vi "AlliGator 1-Exp + IRF Fit v2.vi"(0 "Decay":cluster{"t Array":dbl[], "Data Array":dbl[]}, 1 "Optimal Offset Selection Criterion":T2, 5 "IRF":cluster{"t Array":dbl[], "IRF Array":dbl[]}, 7 "Fit Options":T12={"Show Fit Residuals"=TRUE, "Fit Model"=enum."1-Exponential", "Residual Type"=enum."Standard", "Max Decay Percentile"=0.0, "Min Decay Percentile"=0.0, "Show Full Decay"=TRUE, "Weights"=enum."Unweighted", "Fitting Method"=enum."Least Square", "Compute Parameter Uncertainties"=TRUE, "Periodic Boundaries"=TRUE, "Model Calculation"=enum."Simulation", "Period"=1.2500000000000001e-08, "Termination Criteria"={"Max Iterations"=1000, "Max Function Calls"=0, "Max Time"=1000.0, "Function Tolerance"=1e-06, "Parameter Tolerance"=1e-06, "Gradient Tolerance"=0.0, "Min Lambda"=1e-06, "Max Lambda"=1e-06, "Initial Tick Count"=0}, "Offset Resolution"=1.2500000000000001e-08, "Use Local IRF"=TRUE, "Fitting Algorithm"=enum."Levenberg-Marquardt", "Show Confidence Interval "=TRUE, "Confidence Level"=95.0} {"Confidence Level" min=0.0 max=100.0; "Offset Resolution" min=0.0; "Period" min=0.0; "Min Decay Percentile" min=0.0 max=1.0; "Max Decay Percentile" min=0.0 max=100.0}, 11 "error in (no error)":errorcluster, 12 "parameter bounds":T11) -> (4 "Fit Plots":T1, 8 "Fit Output":T4={"best nonlinear fit"=[], "best fit parameters"=[], "R^2"=0.0, "RMSE"=0.0, "error out"={"status"=FALSE, "code"=0, "source"=""}, "Fitting Method"=enum."Least Square", "number of function calls"=0, "number of iterations"=0, "covariance"=[], "Chi 2"=0.0, "DOF"=0, "Fit Convergence Criterion"=enum."Continue", "Fitting Algorithm"=enum."Levenberg-Marquardt", "Weighted Fit"=enum."Unweighted", "Gradient"=0.0, "|Delta Chi 2|"=0.0, "|Delta Chi 2|/Chi 2"=0.0, "Max |Delta a| /|a|"=0.0, "Lambda"=-1.0, "RSS"=0.0, "AIC"=0.0, "BIC"=0.0, "Max number of function calls"=0, "Max number of iterations"=0, "IRF"={"X Array"=[], "Y Array"=[]}, "IRF Normalization Factor"=0.0, "Decay Normalization Factor"=0.0, "Number of offset fits"=0, "Weighted Chi2"=-1.0, "Unweighted Chi2"=-1.0}, 10 "Delta Best Fit Parameters":dbl[](array[numeric]), 13 "Guess Parameters Options":T3=enum."User-provided (normalized)", 14 "Guess Parameters":dbl[](array[numeric]), 15 "error out":errorcluster)   [LabVIEW 2021, in "AlliGator Decay Fit.lvlib"]
doc: "Legacy code for 1-Exp decay fit."
uses:
  AlliGator Decay Fit.lvlib
  Fits/IRF(X)PSED/Decay Fit Options v4.ctl
  Fits/Decay Convolution/Decay Model.ctl
  Fits/Residual Type.ctl
  Fits/IRF(X)PSED/Fit Weights Type v2.ctl
  Fits/Non-linear Fitting Method v2.ctl
  Fits/Fit Calculation Method.ctl
  Fits/Non-linear Fitting Algorithm.ctl
  Fits/Non-linear Fit Output v4.ctl
  Fits/Nonlinear Fit Method.ctl
  <vilib>/Analysis/Matrix/Datatypes/RealMatrix.ctl
  Fits/Convergence Criteria.ctl
  Graphs/XY Graph/XY Graph Plot Data.ctl
  AlliGator Guess Parameters Options.ctl
  Fits/Optimal Offset Selection Criterion.ctl
  Fits/Fit Plots.ctl
  Settings/AlliGator Settings List.ctl
  Fits/Decay Convolution/Fit Control Data.ctl
  Globals, Variables, Constants/AlliGator Variables List.ctl
  Fits/Decay Convolution/LM model function and gradient (1-Exp, Convolved) v2.vi
  Phasor/Phasor Abort Parallel Computation.vi
  Fits/Decay Convolution/LM model function and gradient (1-Exp, Convolved, Periodic) v3.vi
  Fits/Decay Convolution/LM model function and gradient (1-Exp, Gated, Periodic).vi
  <vilib>/Utility/error.llb/Error Cluster From Error Code.vi
  Fits/Abort Fit Global.vi
  <vilib>/ErrorRing/Error Ring.xnode
  Time/Time.lvlib
  Fits/Fits.lvlib
  Settings/AlliGator Settings.lvlib
  Phasor/Phasor.lvlib
  Globals, Variables, Constants/AlliGator Globals, Variables & Constants.lvlib
  Error/Error.lvlib
  Graphs/XY Graph/XY Graph Add-Ons.lvlib
  <vilib>/Analysis/Matrix/NI_Matrix.lvlib
panel:
  out "CPU (s)":dbl
  out "XY Graph":T17(graph)
  # "Offset\nBaseline\nAmplitude\nLifetime"
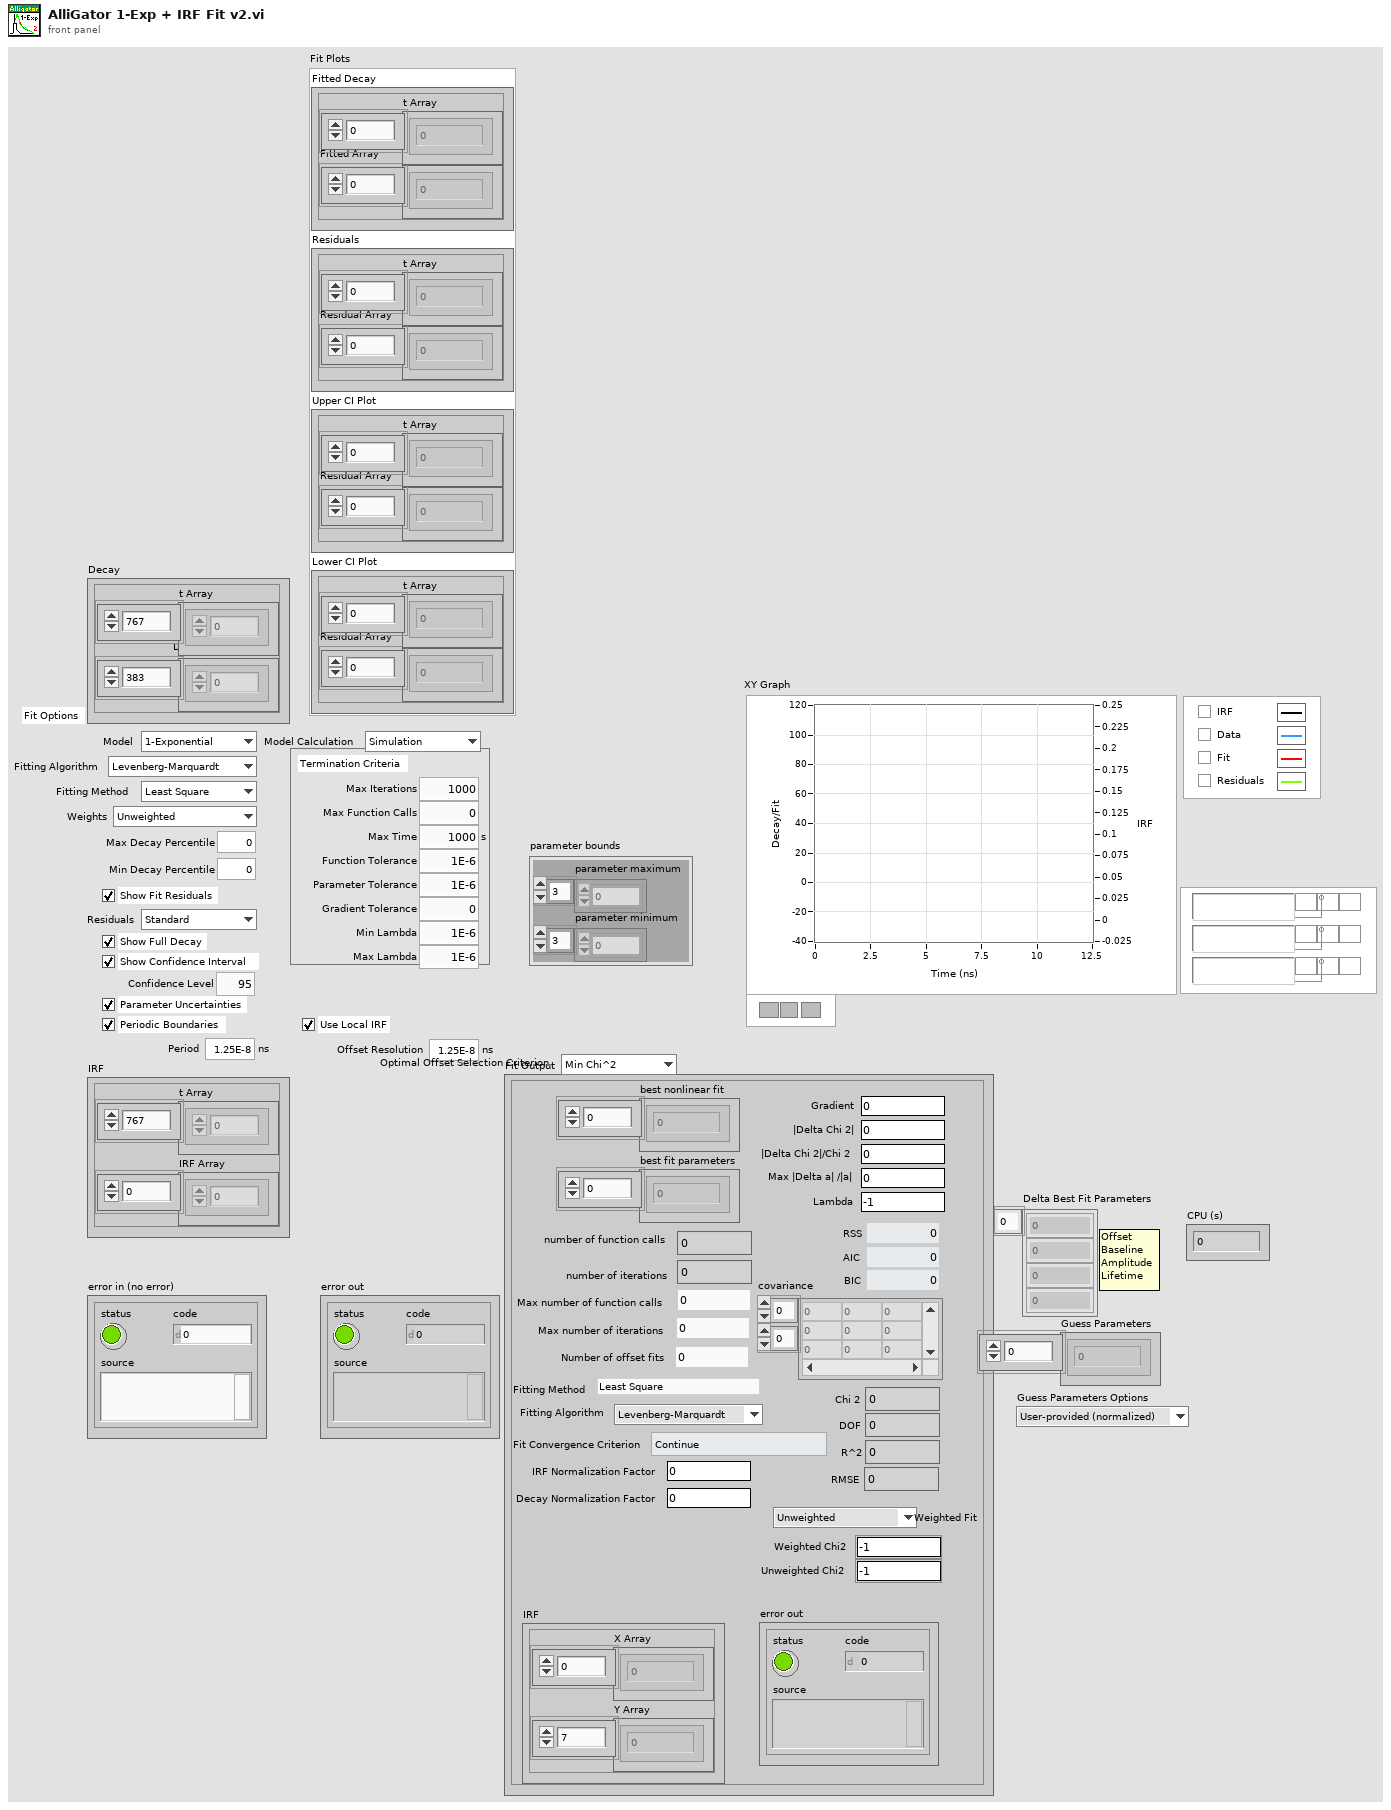
[diagram p1: front panel]
types:
  T1 = typedef "Fits.lvlib/Fit Plots.ctl" = cluster{"Fitted Decay":cluster{"t Array":dbl[], "Fitted Array":dbl[]}, "Residuals":cluster{"t Array":dbl[], "Residual Array":dbl[]}, "Upper CI Plot":cluster{"t Array":dbl[], "Residual Array":dbl[]}, "Lower CI Plot":cluster{"t Array":dbl[], "Residual Array":dbl[]}}
  T2 = typedef "Fits.lvlib/Optimal Offset Selection Criterion.ctl" = enum16{"Min Chi^2", "Max R^2"}
  T3 = typedef "AlliGator Decay Fit.lvlib/AlliGator Guess Parameters Options.ctl" = enum16{"Numerically estimated", "User-provided", "User-provided (normalized)", "Last valid fitted parameters"}
  T4 = typedef "Fits.lvlib/Non-linear Fit Output v4.ctl" = cluster{"best nonlinear fit":dbl[], "best fit parameters":dbl[], "R^2":dbl, "RMSE":dbl, "error out":errorcluster, "Fitting Method":T5, "number of function calls":i32, "number of iterations":i32, "covariance":T6, "Chi 2":dbl, "DOF":i32, "Fit Convergence Criterion":T7, "Fitting Algorithm":T8, "Weighted Fit":T9, "Gradient":dbl, "|Delta Chi 2|":dbl, "|Delta Chi 2|/Chi 2":dbl, "Max |Delta a| /|a|":dbl, "Lambda":dbl, "RSS":dbl, "AIC":dbl, "BIC":dbl, "Max number of function calls":i32, "Max number of iterations":i32, "IRF":T10, "IRF Normalization Factor":dbl, "Decay Normalization Factor":dbl, "Number of offset fits":i32, "Weighted Chi2":dbl, "Unweighted Chi2":dbl}
  T5 = typedef "Fits.lvlib/Nonlinear Fit Method.ctl" = enum16{"Least Square", "Least Absolute Residual", "Bisquare", "MLE"}
  T6 = typedef "NI_Matrix.lvlib/RealMatrix.ctl" = dbl[][]
  T7 = typedef "Fits.lvlib/Convergence Criteria.ctl" = enum16{"Continue", "Tolerances Exceeded", "Max Time Exceeded", "Max Iterations Exceeded", "Max Function Evaluations Exceeded", "Scale Range Exceeded"}
  T8 = typedef "Fits.lvlib/Non-linear Fitting Algorithm.ctl" = enum16{"Levenberg-Marquardt", "Trust-Region Dogleg"}
  T9 = typedef "Fits.lvlib/Fit Weights Type v2.ctl" = enum16{"Unweighted", "1/Variance (Neyman)", "1/Variance (Pearson)", "Best of All"}
  T10 = typedef "XY Graph Add-Ons.lvlib/XY Graph Plot Data.ctl" = cluster{"X Array":dbl[], "Y Array":dbl[]}
  T11 = cluster{"parameter minimum":dbl[], "parameter maximum":dbl[]}
  T12 = typedef "Fits.lvlib/Decay Fit Options v4.ctl" = cluster{"Show Fit Residuals":bool, "Fit Model":T13, "Residual Type":T14, "Max Decay Percentile":dbl, "Min Decay Percentile":dbl, "Show Full Decay":bool, "Weights":T9, "Fitting Method":T15, "Compute Parameter Uncertainties":bool, "Periodic Boundaries":bool, "Model Calculation":T16, "Period":dbl[unit], "Termination Criteria":cluster{"Max Iterations":i32, "Max Function Calls":i32, "Max Time":dbl[unit], "Function Tolerance":dbl, "Parameter Tolerance":dbl, "Gradient Tolerance":dbl, "Min Lambda":dbl, "Max Lambda":dbl, "Initial Tick Count":u32}, "Offset Resolution":dbl[unit], "Use Local IRF":bool, "Fitting Algorithm":T8, "Show Confidence Interval ":bool, "Confidence Level":dbl}
  T13 = typedef "Fits.lvlib/Decay Model.ctl" = enum16{"1-Exponential", "2-Exponentials"}
  T14 = typedef "Fits.lvlib/Residual Type.ctl" = enum16{"Standard", "Normalized", "Reduced"}
  T15 = typedef "Fits.lvlib/Non-linear Fitting Method v2.ctl" = enum16{"Least Square", "Least Absolute Residual", "Bisquare", "MLE", "-", "Best of All"}
  T16 = typedef "Fits.lvlib/Fit Calculation Method.ctl" = enum16{"Simulation", "Convolution", "Integration"}
  T17 = cluster{"t Array":dbl[], "best nonlinear fit":dbl[]}[]
  T18 = typedef "AlliGator Settings.lvlib/AlliGator Settings List.ctl" = enum16{"GUI:Visible Settings Tab", "GUI:Last Run Version", "Source Image:Use Image Histogram for Contrast", "Source Image:Low Count Pixels Rejection Options", "Source Image:High Count Pixels Rejection Options", "Source Image:Use Image Brightness", "Source Image:Blend Overlay with Image Background", "Source Image:Use Fixed ROI Diameter", "Source Image:ROI Diameter", "Source Image:ROI Center Color", "Source Image:Peak Threshold", "Source Image:Intensity Threshold", "Source Image:Image Binning Options", "Source Image:Image Smoothing Options", "Source Image:Image Histogram Active", "Source Image:Invert Binary Mask", "Source Image:Hot Pixel Removal", "Source Image:Overlay Analyzed ROI Center", "Source Image:Auto-Adjust Contrast", "Source Image:Histogram Lower Percentile", "Source Image:Histogram Upper Percentile", "Source Image:Save Source Image", "Source Image:Scale Bar Options", "Source Image:Image Resolution (Pixel Size)", "Source Image:Flatfield Correction", "Source Image:Show Dead Left Columns Correction", "Source Image:Dead Left Columns Correction", "Source Image:Image Pre-Processing Operations Order", "Source Image:Overlay ROI Median", "Source Image:Median Overlay Color", "Data Information:Gate Width", "Data Information:Nanotime Gate Separation", "Data Information:Macrotime Gate Separation", "Data Information:Gate Step", "Data Information:# Gates", "Data Information:Gate Image Exposure", "Data Information:Gate Image Integration", "Data Information:Gates to Skip", "Data Information:Gates to Keep", "Data Information:Define Gates to", "Data Information:Channel Name", "Data Information:Available Channel Names", "Data Information:Channel Arithmetic", "Data Information:Background File Subtraction", "Data Information:Background File", "Data Information:Background Scaling Factor", "Data Information:Background Pile-up Correction", "Data Information:Background Pixel Well Capacity", "Data Information:Laser Period", "Data Information:SYNC Period", "Data Information:Pile-up Correction", "Data Information:Pixel Well Capacity", "Data Information:Dataset Scaling Factor", "Fluorescence Decay_Decay Pre-Processing:Reverse Gates", "Fluorescence Decay_Decay Pre-Processing:Verbose Decay Pre-Processing", "Fluorescence Decay_Decay Pre-Processing:Use Decay Pre-Processing", "Fluorescence Decay_Decay Pre-Processing:Background Subtraction", "Fluorescence Decay_Decay Pre-Processing:Background Definition Range", "Fluorescence Decay_Decay Pre-Processing:Baseline Subtraction Method", "Fluorescence Decay_Decay Pre-Processing:Decay Pre-Processing Operations Order", "Fluorescence Decay_Decay Pre-Processing:Smoothing Parameter", "Fluorescence Decay_Decay Pre-Processing:Shift Decay", "Fluorescence Decay_Decay Pre-Processing:Decay Shift Parameters", "Fluorescence Decay_Decay Pre-Processing:Fold Decay", "Fluorescence Decay_Decay Pre-Processing:# Folds", "Fluorescence Decay_Decay Pre-Processing:1-Normalize Decay", "Fluorescence Decay_Decay Pre-Processing:[0-1]-Normalize Decay", "Fluorescence Decay_Decay Pre-Processing:Smoothen Decay", "Fluorescence Decay_Decay Pre-Processing:Extrapolate Decay", "Fluorescence Decay_Decay Pre-Processing:Use Periodicity", "Fluorescence Decay_Decay Pre-Processing:Use Cursors", "Fluorescence Decay_Decay Pre-Processing:Tail Fraction", "Fluorescence Decay_Decay Pre-Processing:Head Fraction", "Fluorescence Decay_Decay Pre-Processing:Additional Points", "Fluorescence Decay_Decay Pre-Processing:Straighten Decay", "Fluorescence Decay_Decay Pre-Processing:Constant Background", "Fluorescence Decay_Decay Pre-Processing:Pixel-Normalize Decay", "Fluorescence Decay_Advanced Analysis:Extract IRF instead of Decay", "Fluorescence Decay_Advanced Analysis:IRF Extraction Options", "Fluorescence Decay_Advanced Analysis:IRF Optimization Options", "Fluorescence Decay_Advanced Analysis:Square Pulse Options", "Fluorescence Decay_Advanced Analysis:IRF Order", "Fluorescence Decay_Advanced Analysis:IRF Time Constants", "Fluorescence Decay_Advanced Analysis:Wavelet Analysis Options", "Fluorescence Decay_Advanced Analysis:Average Lifetime Options", "Fluorescence Decay_Fit Options:Fit Options", "Fluorescence Decay_Fit Options:Use Legacy Fitting Approach", "Fluorescence Decay_Fit Options:Use Data Information Laser Period", "Fluorescence Decay_Fit Parameters:Displayed Fit Parameters", "Fluorescence Decay_Fit Parameters:Fit Parameter Constraints", "Fluorescence Decay_Fit Parameters:Export Tabulated Results", "Fluorescence Decay_Fit Parameters:MLE Baseline Offset Type", "Fluorescence Decay_Fit Parameters:MLE Baseline Offset", "Fluorescence Decay_Fit Parameters:Guess Parameter Names", "Fluorescence Decay_Fit Parameters:Guess Parameter Values", "Fluorescence Decay_Fit Parameters:Guess Parameters Options", "Fluorescence Decay_Fit Parameters:Optimal Offset Selection Criterion", "Fluorescence Decay_Styles:Show Last Decay Only", "Fluorescence Decay_Styles:Decay Graph Color Array", "Fluorescence Decay:Decay Graph Active", "Fluorescence Decay Statistics:Min Peak Value", "Fluorescence Decay Statistics:Reject Low Decay Peak Pixels", "Fluorescence Decay Statistics:Reject High Decay Peak Pixels", "Fluorescence Decay Statistics:Max Peak Value", "Time Traces:Use File Timestamp", "Time Traces:Time Step", "Time Traces:Use Intensity Correction File", "Time Traces:Intensity Correction File", "Phasor Plot:Phasor Plot Smoothing Options", "Phasor Plot:Phasor Plot Size", "Phasor Plot:Phasor Plot Graphics Options", "Phasor Plot:Cumulative Phasor Plot", "Phasor Plot:Use Phasor Brightness", "Phasor Plot:Blend Overlay with Phasor Background", "Phasor Plot:Save Phasor Plot", "Phasor Plot:Show References", "Phasor Plot:Phasor Ratio Decay Range", "Phasor Plot:Exponential Fading", "Phasor Plot:Phasor Ratio Reference Colors", "Phasor Plot:Reference Radius", "Phasor Plot:Show Color Map Vertices", "Phasor Plot:Phasor Plot Active", "Phasor Plot:Phasor Ratio Color Map Type", "Phasor Plot:Phasor Ratio Color Map", "Phasor Plot:Phasor Ratio Display Range", "Phasor Plot:Selected Image ROI(s)", "Phasor Plot:All Image ROIs", "Phasor Plot:Selected Phasor Plot ROI(s)", "Phasor Plot:All Phasor Plot ROIs", "Phasor Plot:Phasor Ratio Color-Coded Quantity", "Phasor Plot:Store Phasor Harmonics", "Phasor Plot:Draw Reference Segment", "Phasor Plot:User-Defined Quantity", "Phasor Plot:Color Scale High Color", "Phasor Plot:Color Scale Low Color", "Phasor Plot:Intensity-weighted Phasor Plot", "Phasor Graph:Phasor Frequency", "Phasor Graph:Phasor Ratio Type", "Phasor Graph:Pixel-level Phasor Computation", "Phasor Graph:Save Phasor Graph", "Phasor Graph:Phasor Graph Active", "Phasor Graph:Phasor SDV Options", "Phasor Graph:Intensity-weighted Phasor Graph", "Phasor Graph:Define Shortest Lifetime as", "Phasor Calibration:Use Backup Calibration if needed", "Phasor Calibration:Backup Calibration Type", "Phasor Calibration:Calibration Type", "Phasor Calibration:Calibration Lifetime", "Phasor Calibration:Calibration Map Algorithm", "Single-Exponential Phasor Locus (SEPL):Gate Parameters", "Single-Exponential Phasor Locus (SEPL):User-defined Gate", "Single-Exponential Phasor Locus (SEPL):User-defined IRF", "Single-Exponential Phasor Locus (SEPL):Phasor Parameters", "Single-Exponential Phasor Locus (SEPL):Decay & IRF Parameters", "Single-Exponential Phasor Locus (SEPL):Display Parameters", "Lifetime Analysis:Decay Analysis Parameters", "Lifetime Analysis:Lifetime Map Active", "Plugins:Python Settings", "Miscellaneous:Verbose Mode", "Miscellaneous:Beep after Script", "Miscellaneous:Saved Image File Format", "Miscellaneous:Exported Gate Image Settings", "Miscellaneous:Include Loading in Timing", "Miscellaneous:Verbose Settings Mode", "Miscellaneous:Histogram Options", "Miscellaneous:Beep on Error", "Miscellaneous:# Logical Processors Used", "Miscellaneous:ROI Description Max Characters", "Miscellaneous:Verbose Error Mode", "Miscellaneous:Transparent Mask Color"}
  T19 = typedef "Fits.lvlib/Fit Control Data.ctl" = cluster{"IRF":T10, "Laser Period":dbl, "SYNC Period":dbl}
  T20 = typedef "Fits.lvlib/Decay Fit Parameters In List.ctl" = enum16{"Offset", "Baseline", "A_1", "tau_1", "A_2", "tau_2"}
  T21 = typedef "Fits.lvlib/Fit Results (statistics).ctl" = cluster{"Chi2/DOF":dbl, "R2":dbl, "RMSE":dbl, "Fitting Method":T15, "Fitting Algorithm":T8}
  T22 = typedef "AlliGator Globals, Variables & Constants.lvlib/AlliGator Variables List.ctl" = enum16{"---- GUI ----", "GUI:Initialization Status", "GUI:State Indicators Refnum", "GUI:Original AlliGator Menu Items", "GUI:Current Action Loop State", "GUI:Script in progress", "GUI:Playback", "GUI:Loop Playback", "GUI:Search ROI Used", "GUI:Search ROI", "Decay Graph Max Legend Size", "Intensity Graph Max Legend Size", "Decay Statistics Graph Max Legend Size", "Phasor Graph Max Legend Size", "Phasor Ratio Graph Max Legend Size", "Lifetime Graph Max Legend Size", "---- Files ----", "Files:Export Dataset Frames as Individual Files", "Files:Show Batch Export Help Balloons", "Files:Frames in Dataset", "Files:ptu File Frame Start Indices", "Files:Current Frame in Dataset", "Files:Current Frame Timestamp", "Files:Dataset Loaded", "Files:Dataset Metadata", "Files:Dataset Channel", "Files:Dataset Data Description", "Files:Background Dataset Metadata", "Files:Background Dataset Channel", "Files:Background Dataset Data Description", "Files:Background File Subtraction", "Files:Background File Path", "Files:Background File Pile-up Correction", "Files:Background File Pixel Well Capacity", "Files:Background File Scaling Factor", "Files:Current Dataset Load Settings", "Files:Dataset Path", "Files:ICCD-specific Information", "Files:Macrotime Gate Separation", "------ Python Plugins ------", "Python Plugins:Information", "Python Plugins:Python Session", "Python Plugins:Valid Python Session?", "---- Source Image ----", "Source Image:ROIs", "Source Image:Current ROI", "Source Image:ROI Event Refnum", "X_Source Image:Display Range", "X_Source Image:Palette Information", "X_Source Image:Type of Displayed Image", "X_Time Gate Slider", "Source Image:Palette List", "Source Image:Scale", "Source Image:ROI Overlay Color", "Source Image:Overlay to Erase", "Source Image:Is Displayed Image Accumulated", "Source Image:White Light Image Modified", "Source Image:Mask Image Modified", "---- Image Profile Window ----", "Image Profile:Window Event Refnum", "Image Profile:IntensityType", "Image Profile:Intensity Average Type", "Image Profile:Intensity-weighted SDV", "Image Profile:Box Profile Type", "Image Profile:Window Open", "Image Profile:Plotted Fit Parameter", "------ Phasor Graph -------", "Phasor Graph:Show Line", "---- Phasor Plot ---", "Phasor Plot:Parameters Changed", "Phasor Plot:FLI Dataset Modified since last Calculation", "Phasor Harmonics Data", "Selected Phasor Harmonics", "Phasor Harmonic Manager Event Refnum", "Phasor Plot:ROIs", "Phasor Plot:Current ROI", "Phasor Plot:ROI Event Refnum", "Phasor Plot:Image Reference Points", "Phasor Plot:Computed", "Phasor Plot:Palette Information", "Phasor Plot:Palette List", "Phasor Plot:Phasor Ratio Palette Information", "Phasor Plot:Phasor Ratio Palette List", "Phasor Plot:Image Scale", "Phasor Plot:Image Overlay to Erase", "Phasor Plot:Image Elements to Update", "Phasor Plot:Current Calculation Parameters", "Phasor Plot:Current Calibration Options", "Phasor Plot:Reset Cumulated Phasor Plot", "Phasor Plot:Reference 1", "Phasor Plot:Lifetime Reference 1", "Phasor Plot:Reference 1 Frequency", "Phasor Plot:Reference 2", "Phasor Plot:Lifetime Reference 2", "Phasor Plot:Reference 2 Frequency", "---- Decay Analysis ----", "Number of Selected Decays to Fit", "LS Fit Results", "LAR Fit Results", "BS Fit Results", "Last Decay Max - Min", "Best Fit Parameters", "Best Fit Parameter Names", "Actual Size X", "Actual Size Y", "Binning X", "Binning Y", "Actual # Gates", "Dataset Number", "Gates to...", "Gates Skipped", "Gates to keep", "Gate Step", "Gate Separation", "Reversed Gates", "Pile-up Correction", "Pixel Well Capacity", "Background Subtracted", "Background Subtraction Method", "Background Definition Range", "Background File (deprecated)", "Number of Dataset Accumulated", "Array of Accumulated Dataset Paths", "Do Averaged Datasets", "Destination File Path", "Process Plot Target", "Use 1/D as Phasor Frequency", "---- Decay Fit Parameter Map -----", "Decay Fit Parameter Map:Palette Information", "Decay Fit Parameter Map:Palette List", "Decay Fit Parameter Map:X Resolution", "Decay Fit Parameter Map:Y Resolution", "Decay Fit Parameter Map:Use Decay Fit Result Constraints", "Decay Fit Parameter Map:Decay Fit Result Constraints", "Decay Fit Parameter Map:Decay Fit Result Constraints Applied", "---- Parameter Map ----", "Parameter Map:Palette Information", "Parameter Map:Palette List", "------- Local Decay Window ---------", "Local Decay Graph Window:Event Refnum", "Local Decay Graph Window:Use normalized IRF for convolution", "----- Miscellaneous ----", "Misc:Skippable Dialog Windows Status"}
  T23 = cluster{"t Array":dbl[], "best nonlinear fit":dbl[]}
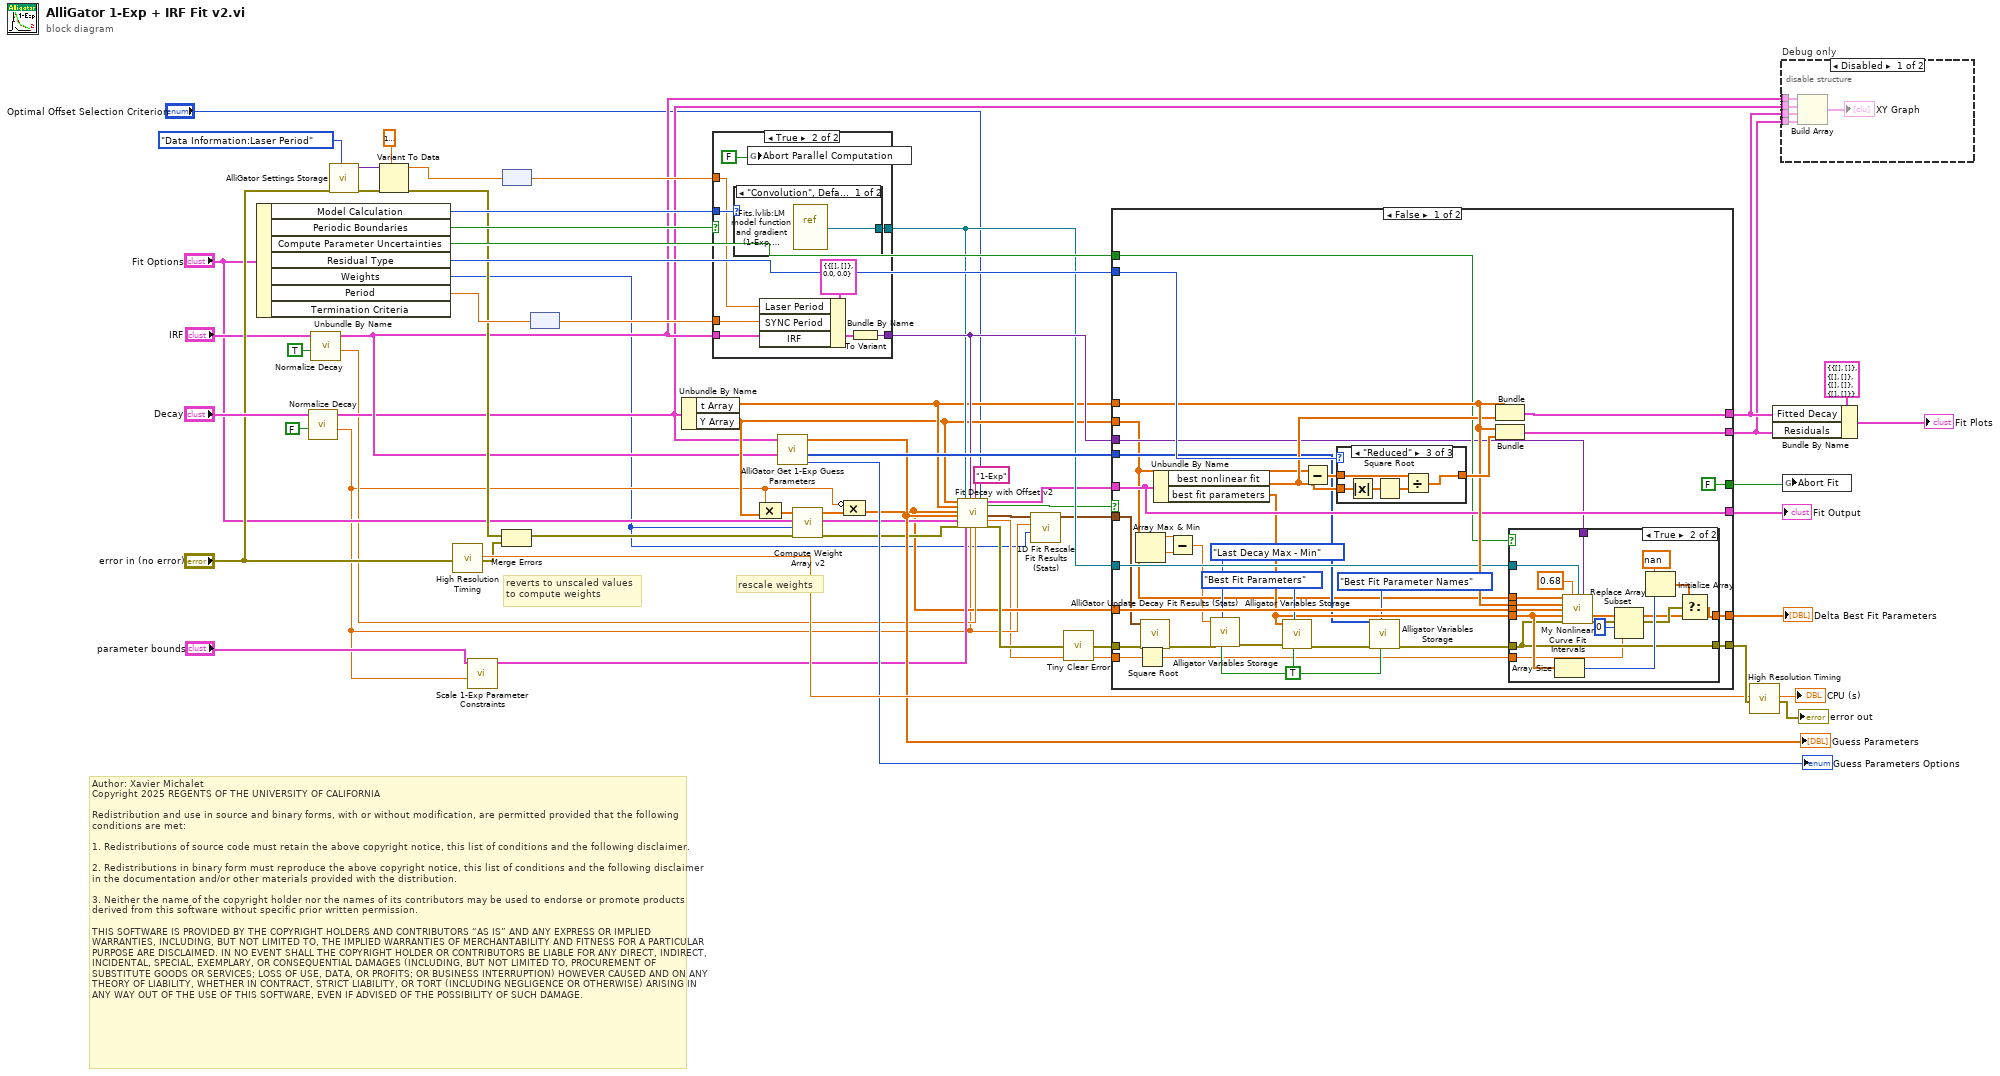
[diagram p0: block diagram]
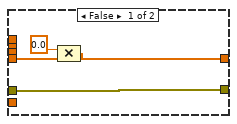
[diagram p3: hidden frame]
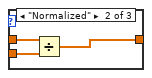
[diagram p5: hidden frame]
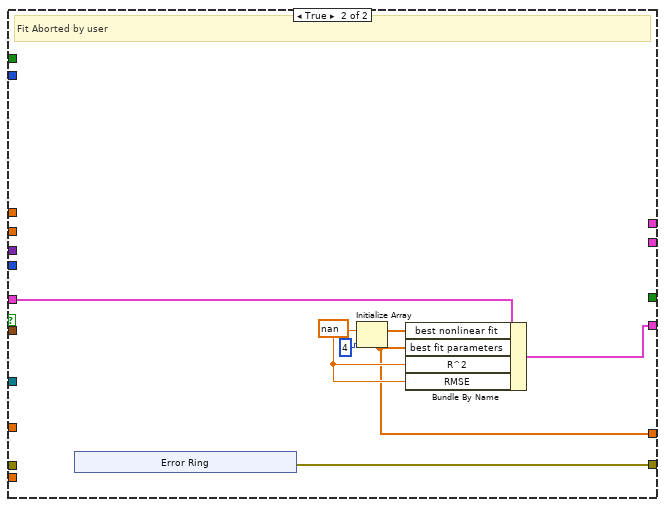
[diagram p6: hidden frame]
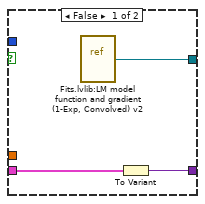
[diagram p7: hidden frame]
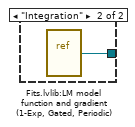
[diagram p8: hidden frame]
diagram:
  # "Author: Xavier Michalet\nCopyright 2025 REGENTS OF THE UNIVERSITY OF CALIFORNIA\n\nRedistribution and use in source and binary forms, with or without modification, are permitted provided that the following conditions are met:\n\n1. Redistributions of source code must retain the above copyright notice, this list of conditions and the following disclaimer.\n\n2. Redistributions in binary form must reproduce the above copyright notice, this list of conditions and the following disclaimer in the documentation and/or other materials provided with the distribution.\n\n3. Neither the name of the copyright holder nor the names of its contributors may be used to endorse or promote products derived from this software without specific prior written permission.\n\nTHIS SOFTWARE IS PROVIDED BY THE COPYRIGHT HOLDERS AND CONTRIBUTORS “AS IS” AND ANY EXPRESS OR IMPLIED WARRANTIES, INCLUDING, BUT NOT LIMITED TO, THE IMPLIED WARRANTIES OF MERCHANTABILITY AND FITNESS FOR A PARTICULAR PURPOSE ARE DISCLAIMED. IN NO EVENT SHALL THE COPYRIGHT HOLDER OR CONTRIBUTORS BE LIABLE FOR ANY DIRECT, INDIRECT, INCIDENTAL, SPECIAL, EXEMPLARY, OR CONSEQUENTIAL DAMAGES (INCLUDING, BUT NOT LIMITED TO, PROCUREMENT OF SUBSTITUTE GOODS OR SERVICES; LOSS OF USE, DATA, OR PROFITS; OR BUSINESS INTERRUPTION) HOWEVER CAUSED AND ON ANY THEORY OF LIABILITY, WHETHER IN CONTRACT, STRICT LIABILITY, OR TORT (INCLUDING NEGLIGENCE OR OTHERWISE) ARISING IN ANY WAY OUT OF THE USE OF THIS SOFTWARE, EVEN IF ADVISED OF THE POSSIBILITY OF SUCH DAMAGE."
  # "rescale weights"
  # "reverts to unscaled values to compute weights"
  n1 = Unbundle By Name("Fit Options") -> ("Model Calculation"=w44:T16, "Periodic Boundaries"=w51:bool, "Compute Parameter Uncertainties"=w52:bool, "Residual Type"=w55:T14, "Weights"=w1:T9, "Period"=w41:dbl[unit])  [unwired: 1 out]
  n2 = call "Normalize Decay.vi"("IRF (F)"=FALSE, "Decay"="Decay") -> ("Normalization Factor"=w8:dbl, "Normalized Decay"=w22:cluster{"t Array":dbl[], "Y Array":dbl[]})  [unwired: 7 in, 1 out]
  n3 = call "Normalize Decay.vi"("IRF (F)"=TRUE, "Decay"="IRF") -> ("Normalization Factor"=w11:dbl, "Normalized Decay"=w23:cluster{"t Array":dbl[], "Y Array":dbl[]})  [unwired: 7 in, 1 out]
  n4 = call "AlliGator Settings Storage.vi"("AlliGator Settings List"=AlliGator_Settings_List."Data Information:Laser Period", "Error In"="error in (no error)") -> ("Error Out"=w48:errorcluster, "Variant Data out"=w49:variant)  [unwired: 8 in]
  n5 = Variant To Data(error in=w48, type=dbl[unit] 1e-09 ("New"), Variant=w49) -> (data=w46:dbl[unit], error out=w29:errorcluster)
  n6 = call "High Resolution Timing.vi"("Error In"="error in (no error)") -> ("elapsed (relative) seconds"=w57:dbl, "Error Out"=w31:errorcluster)  [unwired: 16 in, 1 out]
  n7 = call "Scale 1-Exp Parameter Constraints.vi"("Normalization Factor"=w8, "parameter bounds in"="parameter bounds") -> ("parameter bounds out"=w15:T11)  [unwired: 9 in]
  n8 = Merge Errors(w29, w31) -> (w28:errorcluster)
  n9 = node(w46) -> (w45:dbl)
  n10 = node(w41) -> (w40:dbl)
  n11 = Unbundle By Name(w22) -> ("t Array"=w37:dbl[], "Y Array"=w34:dbl[])
  n12 = case shown="True" w51 {
    tunnel: [w62 w71] -> w38
    tunnel: w23 -> [w61 w70]
    tunnel: [w60 w68] -> w39
    tunnel: w45 -> [_ w64]
    tunnel: w44 -> [_ w66]
    tunnel: w40 -> [_ w63]
    frame False {
      n13 = vi-ref "Fits.lvlib:LM model function and gradient (1-Exp, Convolved) v2.vi"() -> (w62:refnum<vi>)
      n14 = To Variant(anything=w61) -> (Variant=w60:variant)
    }
    frame True {
      n15 = case shown="\"Convolution\", Default" w66 {
        tunnel: [w72 w73] -> w71
        frame "Convolution", Default {
          n16 = vi-ref "Fits.lvlib:LM model function and gradient (1-Exp, Convolved, Periodic) v3.vi"() -> (w72:refnum<vi>)
        }
        frame "Integration" {
          n17 = vi-ref "Fits.lvlib:LM model function and gradient (1-Exp, Gated, Periodic).vi"() -> (w73:refnum<vi>)
        }
      }
      n18 = global write "Phasor Abort Parallel Computation.vi" "Abort Parallel Computation"(FALSE ("Abort Parallel Computation")) -> ()
      n19 = Bundle By Name(cluster=T19 {"IRF"={"X Array"=[], "Y Array"=[]}, "Laser Period"=0.0, "SYNC Period"=0.0}, "Laser Period"=w64, "SYNC Period"=w63, "IRF"=w70) -> (w69:T19)
      n20 = To Variant(anything=w69) -> (Variant=w68:variant)
    }
  }
  n21 = Compound Arithmetic op=MULTIPLY(w8, w34) -> (w10:dbl[])
  n22 = call "AlliGator Get 1-Exp Guess Parameters.vi"("IRF"=w23, "Decay"=w22) -> ("Guess Parameters Type"=→"Guess Parameters Options":T3, "Guess Parameters Names"=w43:T20[], "Guess Parameters"=w36:dbl[])  [unwired: 7 in]
  "Guess Parameters" <- w36
  n23 = call "Compute Weight Array v2.vi"("Error In"=w28, "Weighted Fit"=w1, "Data Array"=w10) -> ("Error Out"=w30:errorcluster, "Weight Array"=w35:dbl[])  [unwired: 7 in]
  n24 = Compound Arithmetic op=MULTIPLY(invert w8, w35) -> (w9:dbl[])
  n25 = call "Fit Decay with Offset v2.vi"("Y Array"=w34, "X Array"=w37, "Weights"=w9, "Initial Parameters"=w36, "Decay Fit Options"="Fit Options", "error in (no error)"=w30, "f(x,a)"=w38, "parameter bounds"=w15, "Data"=w39, "Decay Normalization Factor"=w8, "Model Name"="1-Exp", "IRF Normalization Factor"=w11, "Optimal Offset Selection Criterion"="Optimal Offset Selection Criterion") -> ("Fit Output"=w16:T4, "Fit Aborted?"=w27:bool, "Fit Results (Stats)"=w18:T21[], "C_00"=w7:dbl, "error out"=w25:errorcluster)  [unwired: 2 in]
  n26 = call "1D Fit Rescale Fit Results (Stats).vi"("Weighted"=w1, "Normalization Factor"=w8, "Fit Results (Stats) in"=w18) -> ("Fit Results (Stats) out"=w17:T21[])  [unwired: 8 in]
  n27 = call "Tiny Clear Error.vi"("Error In"=w25) -> ("no Error Out"=w24:errorcluster)  [unwired: 8 in]
  n28 = case shown="False" w27 {
    tunnel: [w106 _] -> w3
    tunnel: [w105 w141] -> w59
    tunnel: [w104 w137] -> w58
    tunnel: [w103 _] -> w2
    tunnel: w55 -> [w102 _]
    tunnel: w37 -> [w99 _]
    tunnel: w38 -> [w98 _]
    tunnel: w34 -> [w81 _]
    tunnel: w9 -> [w97 _]
    tunnel: w16 -> [w95 w140]
    tunnel: [w95 w139] -> w53
    tunnel: w52 -> [w94 _]
    tunnel: w39 -> [w93 _]
    tunnel: w43 -> [w87 _]
    tunnel: w24 -> [w86 _]
    tunnel: w17 -> [w77 _]
    tunnel: [FALSE ("Abort Fit") _] -> w13
    tunnel: w7 -> [w75 _]
    frame False {
      w83 = TRUE ("Get(F)/Set")
      n29 = Array Max & Min(array=w81) -> (max value=w80:dbl, min value=w79:dbl)  [unwired: 2 out]
      n30 = Square Root(x=w75) -> (sqrt(x)=w74:dbl)
      n31 = call "AlliGator Update Decay Fit Results (Stats).vi"("error in (no error)"=w86, "Fit Results"=w77) -> ("error out"=w85:errorcluster)  [unwired: 9 in]
      n32 = Unbundle By Name(w95) -> ("best nonlinear fit"=w96:dbl[], "best fit parameters"=w91:dbl[])
      n33 = Subtract(x=w80, y=w79) -> (x-y=w78:dbl)
      n34 = call "Alligator Variables Storage.vi"("Get(F)/Set"=w83, "AlliGator Variable"=AlliGator_Variables_List."Last Decay Max - Min" ("Alligator Variable"), "Error In"=w85, "Data in"=w78) -> ("Error Out"=w84:errorcluster)  [unwired: 5 in, 2 out]
      n35 = call "Alligator Variables Storage.vi"("Get(F)/Set"=w83, "AlliGator Variable"=AlliGator_Variables_List."Best Fit Parameters" ("Alligator Variable"), "Error In"=w84, "Data in"=w91) -> ("Error Out"=w90:errorcluster)  [unwired: 5 in, 2 out]
      n36 = Subtract(x=w81, y=w96) -> (x-y=w101:dbl[])
      n37 = case shown="\"Reduced\"" w102 {
        tunnel: w101 -> [w128 w131 w136]
        tunnel: [w128 w129 w134] -> w100
        tunnel: w96 -> [_ w130 w135]
        frame "Standard", Default {
        }
        frame "Normalized" {
          n38 = Divide(x=w131, y=w130) -> (x/y=w129:dbl[])
        }
        frame "Reduced" {
          n39 = Absolute Value(x=w135) -> (abs(x)=w133:dbl[])
          n40 = Square Root(x=w133) -> (sqrt(x)=w132:dbl[])
          n41 = Divide(x=w136, y=w132) -> (x/y=w134:dbl[])
        }
      }
      n42 = call "Alligator Variables Storage.vi"("Get(F)/Set"=w83, "AlliGator Variable"=AlliGator_Variables_List."Best Fit Parameter Names" ("Alligator Variable"), "Error In"=w90, "Data in"=w87) -> ("Error Out"=w89:errorcluster)  [unwired: 5 in, 2 out]
      n43 = Bundle("t Array"=w99, "best nonlinear fit"=w96) -> (w106:T23)  [unwired: 1 in]
      n44 = Bundle("t Array"=w99, w100) -> (w103:cluster{"t Array":dbl[], dbl[]})  [unwired: 1 in]
      n45 = case shown="True" w94 {
        tunnel: [w110 w114] -> w105
        tunnel: [w108 w115] -> w104
        tunnel: w99 -> [_ w126]
        tunnel: w98 -> [_ w125]
        tunnel: w97 -> [_ w124]
        tunnel: w93 -> [_ w123]
        tunnel: w91 -> [w109 w121]
        tunnel: w81 -> [_ w122]
        tunnel: w89 -> [w110 w114]
        tunnel: w74 -> [_ w111]
        frame False {
          n46 = Compound Arithmetic op=MULTIPLY(0.0, w109) -> (w108:dbl[])
        }
        frame True {
          n47 = Array Size(array=w121) -> (size(s)=w120:i32)
          n48 = call "My Nonlinear Curve Fit Intervals.vi"("Y"=w122, "confidence level"=0.68, "f(x,a)"=w125, "data"=w123, "X"=w126, "Weight"=w124, "best fit parameters"=w121, "error in (no error)"=w114) -> ("delta best fit parameters"=w116:dbl[], "error out"=w117:errorcluster)  [unwired: 6 in]
          n49 = Replace Array Subset(array=w116, new element=w111, index=0) -> (w113:dbl[])
          n50 = Initialize Array(nan ("element"), w120) -> (w118:dbl[])
          n51 = Select(t=w118, s=w117, f=w113) -> (s? t:f=w115:dbl[])
        }
      }
    }
    frame True {
      w138 = nan ("element")
      # "Fit Aborted by user"
      n52 = xnode "Error Ring"() -> ("error out"=w141:errorcluster)
      n53 = Initialize Array(w138, 4 ("dimension size")) -> (w137:dbl[])
      n54 = Bundle By Name(cluster=w140, "best nonlinear fit"=w137, "best fit parameters"=w137, "R^2"=w138, "RMSE"=w138) -> (w139:T4)
    }
  }
  "Delta Best Fit Parameters" <- w58
  "Fit Output" <- w53
  n55 = call "High Resolution Timing.vi"("relative seconds (NaN)"=w57, "Error In"=w59) -> ("elapsed (relative) seconds"=→"CPU (s)":dbl, "Error Out"=→"error out":errorcluster)  [unwired: 15 in, 1 out]
  n56 = Bundle By Name(cluster=T1 {"Fitted Decay"={"t Array"=[], "Fitted Array"=[]}, "Residuals"={"t Array"=[], "Residual Array"=[]}, "Upper CI Plot"={"t Array"=[], "Residual Array"=[]}, "Lower CI Plot"={"t Array"=[], "Residual Array"=[]}} ("Fit Plots"), "Fitted Decay"=w3, "Residuals"=w2) -> (→"Fit Plots":T1)
  n57 = disable-structure "Debug only" shown="Disabled" {
    disable-tunnel: w23 -> [w151 _]
    disable-tunnel: w22 -> [w150 _]
    disable-tunnel: w3 -> [w149 _]
    disable-tunnel: w2 -> [w148 _]
    frame Disabled {
      n58 = Build Array(w151, w150, w149, w148) -> (→"XY Graph":T17)
    }
    frame Enabled {
    }
  }
  n59 = global write "Abort Fit Global.vi" "Abort Fit"(w13) -> ()
